vi "SendCommand.vi"(8 "error in (no error)":errorcluster, 10 "Command string":string, 11 "InstControl in":refnum<class "InstrControl.lvclass">) -> (0 "error out":errorcluster, 3 "InstControl out":refnum<class "InstrControl.lvclass">)   [LabVIEW 2013, in "InstrControl.lvclass"]
uses:
  InstrControl.lvclass
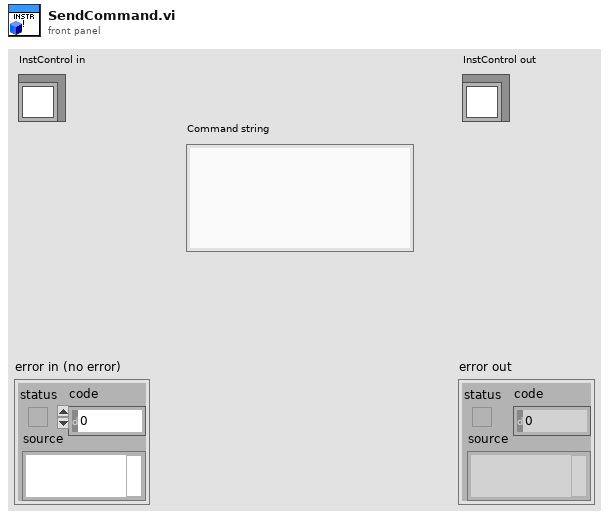
[diagram p1: front panel]
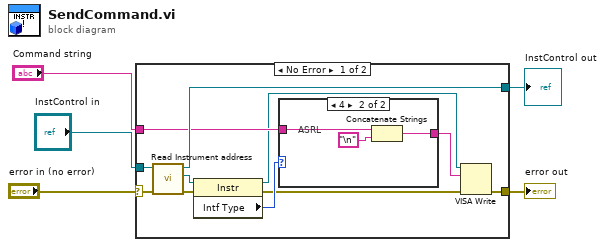
[diagram p0: block diagram]
diagram:
  n1 = case shown="No Error" "error in (no error)" {
    selector: "error in (no error)" -> [w15 w22]
    tunnel: [w13 w22] -> w4
    tunnel: [w16 w21] -> w3
    tunnel: "InstControl in" -> [w14 w21]
    tunnel: "Command string" -> [w10 _]
    frame No Error {
      n2 = call-dynamic "Read Instrument address.vi"("error in (no error)"=w15, "InstControl in"=w14) -> ("error out"=w8:errorcluster, "VISA address"=w12:refnum<visa-resource-name>, "InstControl out"=w16:refnum<class "InstrControl.lvclass">)  [unwired: 7 in]
      n3 = property class="Instr"(reference=w12, error in=w8) -> (reference out=w6:refnum<visa-resource-name>, error out=w7:errorcluster, "Intf Type"=w11:u16)
      n4 = case shown="4" w11 {
        tunnel: [w17 w18] -> w9
        tunnel: w10 -> [w17 w20]
        frame 1, Default {
          # "GPIB"
        }
        frame 4 {
          # "ASRL"
          n5 = Concatenate Strings(w20, "\n") -> (w18:string)
        }
      }
      n6 = VISA Write(VISA resource name=w6, write buffer=w9, error in (no error)=w7) -> (error out=w13:errorcluster)  [unwired: 2 out]
    }
    frame Error {
    }
  }
  "error out" <- w4
  "InstControl out" <- w3
